vi "Tosca-Process Events.vi"(0 "Accum States in":T1[](array[typedef]), 2 "Digital Inputs":T2[](array[typedef]), 5 "state change":bool, 7 "Input Events":T3[](array[typedef])) -> (4 "Accum States out":T1[](array[typedef]), 8 "Events":bool[](array[boolean]))   [LabVIEW 2020]
uses:
  Tosca-Input Event.ctl
  Tosca-Input Criterion.ctl
  epl-vi-lib/Utility VIs/Type Defs/Logic State.ctl
  Typedefs/Tosca-Accumulator.ctl
  Tosca-Digital Input.ctl
  Typedefs/Tosca-Accumulator State.ctl
  epl-vi-lib/Utility VIs/Math VIs/X1000.vi
  Sub VIs/Tosca-Globals.vi
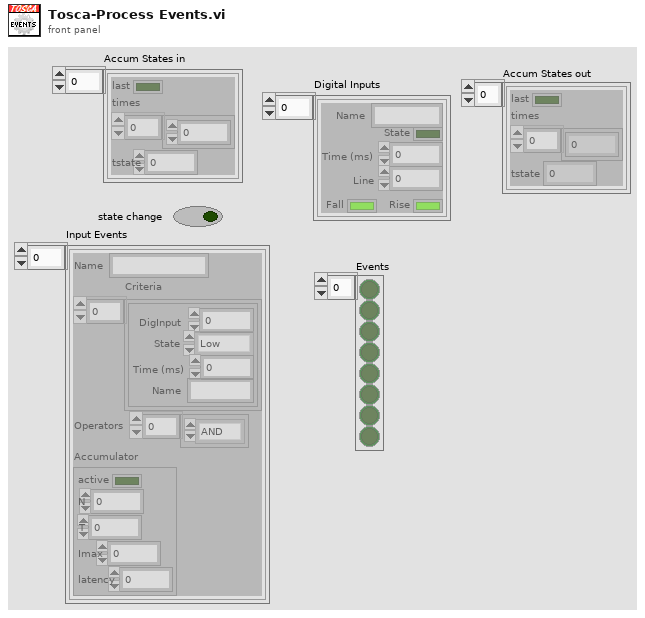
[diagram p1: front panel]
types:
  T1 = typedef "Tosca-Accumulator State.ctl" = cluster{"last":bool, "times":dbl[], "tstate":dbl}
  T2 = typedef "Tosca-Digital Input.ctl" = cluster{"Name":string, "State":bool, "Time (ms)":dbl, "Line":i32, "Rise":bool, "Fall":bool}
  T3 = typedef "Tosca-Input Event.ctl" = cluster{"Name":string, "Criteria":T4[], "Operators":enum16{"AND", "OR"}[], "Accumulator":T6}
  T4 = typedef "Tosca-Input Criterion.ctl" = cluster{"DigInput":i32, "State":T5, "Time (ms)":i32, "Name":string}
  T5 = typedef "Logic State.ctl" = enum16{"Low", "High", "Rising", "Falling"}
  T6 = typedef "Tosca-Accumulator.ctl" = cluster{"active":bool, "N":i32, "T":dbl, "Imax":dbl, "latency":dbl}
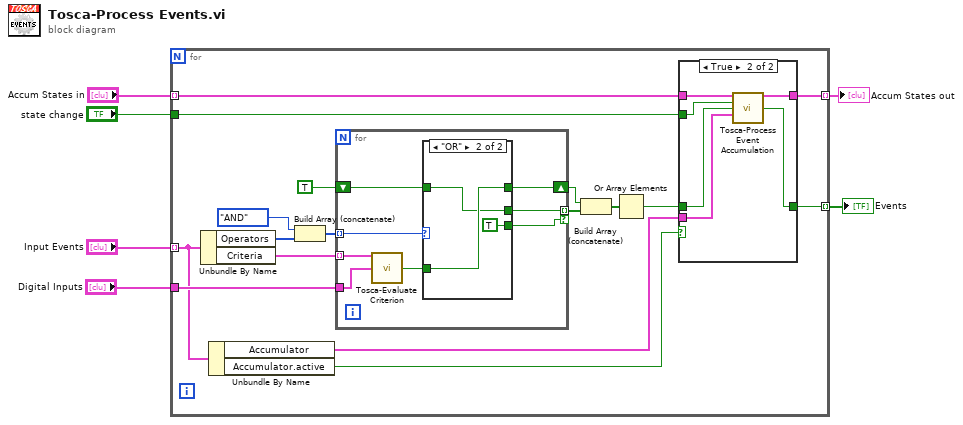
[diagram p0: block diagram]
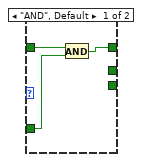
[diagram p3: hidden frame]
diagram:
  n1 = for {
    tunnel: "Digital Inputs" -> [w18]
    tunnel: "Input Events" -> [w14] mode=indexing
    tunnel: [w13] -> w4 mode=indexing
    tunnel: "Accum States in" -> [w9] mode=indexing
    tunnel: [w8] -> w2 mode=indexing
    tunnel: "state change" -> [w7]
    n2 = Unbundle By Name(w14) -> ("Operators"=w22:enum16{"AND", "OR"}[], "Criteria"=w23:T4[])
    n3 = Unbundle By Name(w14) -> ("Accumulator"=w10:T6, "Accumulator.active"=w11:bool)
    n4 = Build Array (concatenate)(enum16{"AND", "OR"}."AND" ("Operator"), w22) -> (w19:enum16{"AND", "OR"}[])
    n5 = for {
      tunnel: w23 -> [w39] mode=indexing
      shift-right: [w34] -> w15
      shift-left: TRUE -> [w35]
      tunnel: w19 -> [w36] mode=indexing
      tunnel: w18 -> [w38]
      tunnel: [w33] -> w16 mode=indexing if=w32
      n6 = call "Tosca-Evaluate Criterion.vi"("Criterion"=w39, "Digital Inputs"=w38) -> ("Criterion met?"=w37:bool)  [unwired: 13 in]
      n7 = case shown="\"OR\"" w36 {
        tunnel: w37 -> [w40 w45]
        tunnel: w35 -> [w42 w44]
        tunnel: [w41 w45] -> w34
        tunnel: [_ w44] -> w33
        tunnel: [_ TRUE] -> w32
        frame "AND", Default {
          n8 = And(x=w42, y=w40) -> (x .and. y?=w41:bool)
        }
        frame "OR" {
        }
      }
    }
    n9 = Build Array (concatenate)(w15, w16) -> (w17:bool[])
    n10 = Or Array Elements(Boolean array=w17) -> (logical OR=w12:bool)
    n11 = case shown="True" w11 {
      tunnel: [w25 w27] -> w13
      tunnel: w12 -> [w25 w28]
      tunnel: w10 -> [_ w29]
      tunnel: w9 -> [w24 w31]
      tunnel: [w24 w30] -> w8
      tunnel: w7 -> [_ w26]
      frame False {
      }
      frame True {
        n12 = call "Tosca-Process Event Accumulation.vi"("accum state in"=w31, "state change"=w26, "Value in"=w28, "Accumulator"=w29) -> ("accum state out"=w30:T1, "Value out"=w27:bool)  [unwired: 10 in]
      }
    }
  }
  "Events" <- w4
  "Accum States out" <- w2
